vi "Generate Randon UUID.vi"(11 "Taille":i32=16) -> (3 "chaîne":string)   [LabVIEW 2020, in "Library Commun.lvlib"]
uses:
  Library Commun.lvlib
panel:
  out "?":i32
  # "c"
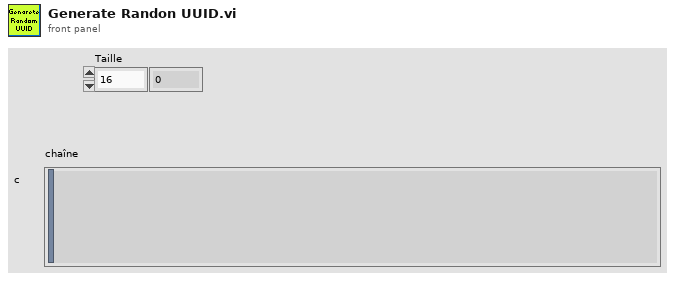
[diagram p1: front panel]
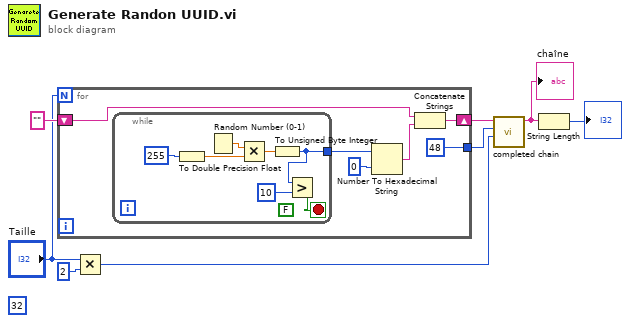
[diagram p0: block diagram]
diagram:
  (unwired) 32 ("longueur")
  n1 = for {
    N: "Taille" -> [_]
    shift-right: [w14] -> w6
    shift-left: "" -> [w13]
    tunnel: [u8 48 ("Combler par")] -> w8
    n2 = while {
      tunnel: [w17] -> w10
      stop <- w15 stop-if-true
      (unwired) FALSE
      n3 = To Double Precision Float(number=u8 255 ("nombre")) -> (double precision float=w19:dbl)
      n4 = Random Number (0-1)() -> (number: 0 to 1=w20:dbl)
      n5 = Multiply(x=w20, y=w19) -> (x*y=w18:dbl)
      n6 = To Unsigned Byte Integer(number=w18) -> (unsigned 8bit integer=w17:u8)
      n7 = Greater?(x=w17, y=u8 10) -> (0:w15:bool)
    }
    n8 = Number To Hexadecimal String(1:u8 0 ("largeur (-)"), 2:w10) -> (0:w9:string)
    n9 = Concatenate Strings(w13, w9) -> (w14:string)
  }
  n10 = Multiply(x="Taille", y=2) -> (x*y=w3:i32)
  n11 = call "completed chain.vi"("longueur"=w3, "Combler par"=w8, "Chaine"=w6) -> ("chaîne"=w2:string)  [unwired: 8 in]
  "chaîne" <- w2
  n12 = String Length(string=w2) -> (length=→"?":i32)
